vi "X-Y-Z-Move-Pro_Api.vi"() -> ()   [LabVIEW 2019]
uses:
  <vilib>/Platform/TimedLoop/XDataNode/timing_clust.ctl
  <vilib>/Platform/TimedLoop/XDataNode/nitl_modes.ctl
  <vilib>/Platform/TimedLoop/XDataNode/wakeup.ctl
  <vilib>/platform/TimedLoop/XDataNode/XDataNode.xnode
  <vilib>/Platform/TimedLoop/XDataNode/XDNodeRunTimeDep.lvlib
panel:
  out "Waveform Chart":cluster{dbl, dbl}(graph)
  in  "Stop":bool
  out "Error Out":errorcluster
  in  "Error In":errorcluster
  in  "加速度":dbl=800.0
  in  "最高速":dbl=1150.0
  in  "X-Y-Z移動":dbl[][](array[numeric])=[[0.0, 0.0, 0.0]]
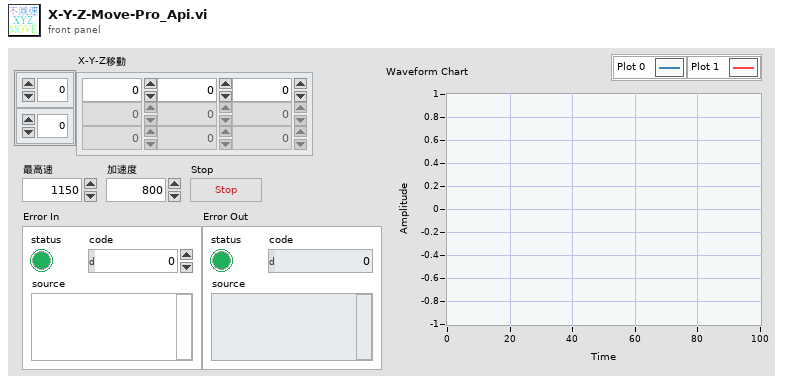
[diagram p1: front panel]
types:
  T1 = typedef "XDNodeRunTimeDep.lvlib/timing_clust.ctl" = cluster{"Expected End [f-1]":u64, "Actual End [f-1]":u64, "Finished Late? [f-1]":bool, "Expected End [i-1]":u64, "Actual End [i-1]":u64, "Finished Late? [i-1]":bool, "Expected Start [i]":u64, "Actual Start [i]":u64, "Expected Start [f]":u64, "Actual Start [f]":u64, "Source Name":string, "Structure Name":string, "Period":i64, "Deadline":i64, "Offset":i64, "Start":i64, "Priority":i32, "Timeout":i32, "Mode":T2, "Wakeup Reason":T3, "Error":errorcluster, "Source Type":string, "Secondary Source Type":string, "Global End Time":u64, "Global Start Time":u64, "Frame Duration":u64, "Iteration Duration":u64, "Assigned CPU":i32, "I/O Scan Engine Mode":u32}
  T2 = typedef "XDNodeRunTimeDep.lvlib/nitl_modes.ctl" = enum32{"No Change", "Process missed periods, maintain original phase", "Discard missed periods, maintain original phase", "Process missed periods, ignore original phase", "Discard missed periods, ignore original phase"}
  T3 = typedef "XDNodeRunTimeDep.lvlib/wakeup.ctl" = enum32{"Normal", "Aborted", "Asynchronous wakeup", "Timing source error", "Timed loop error", "Timeout"}
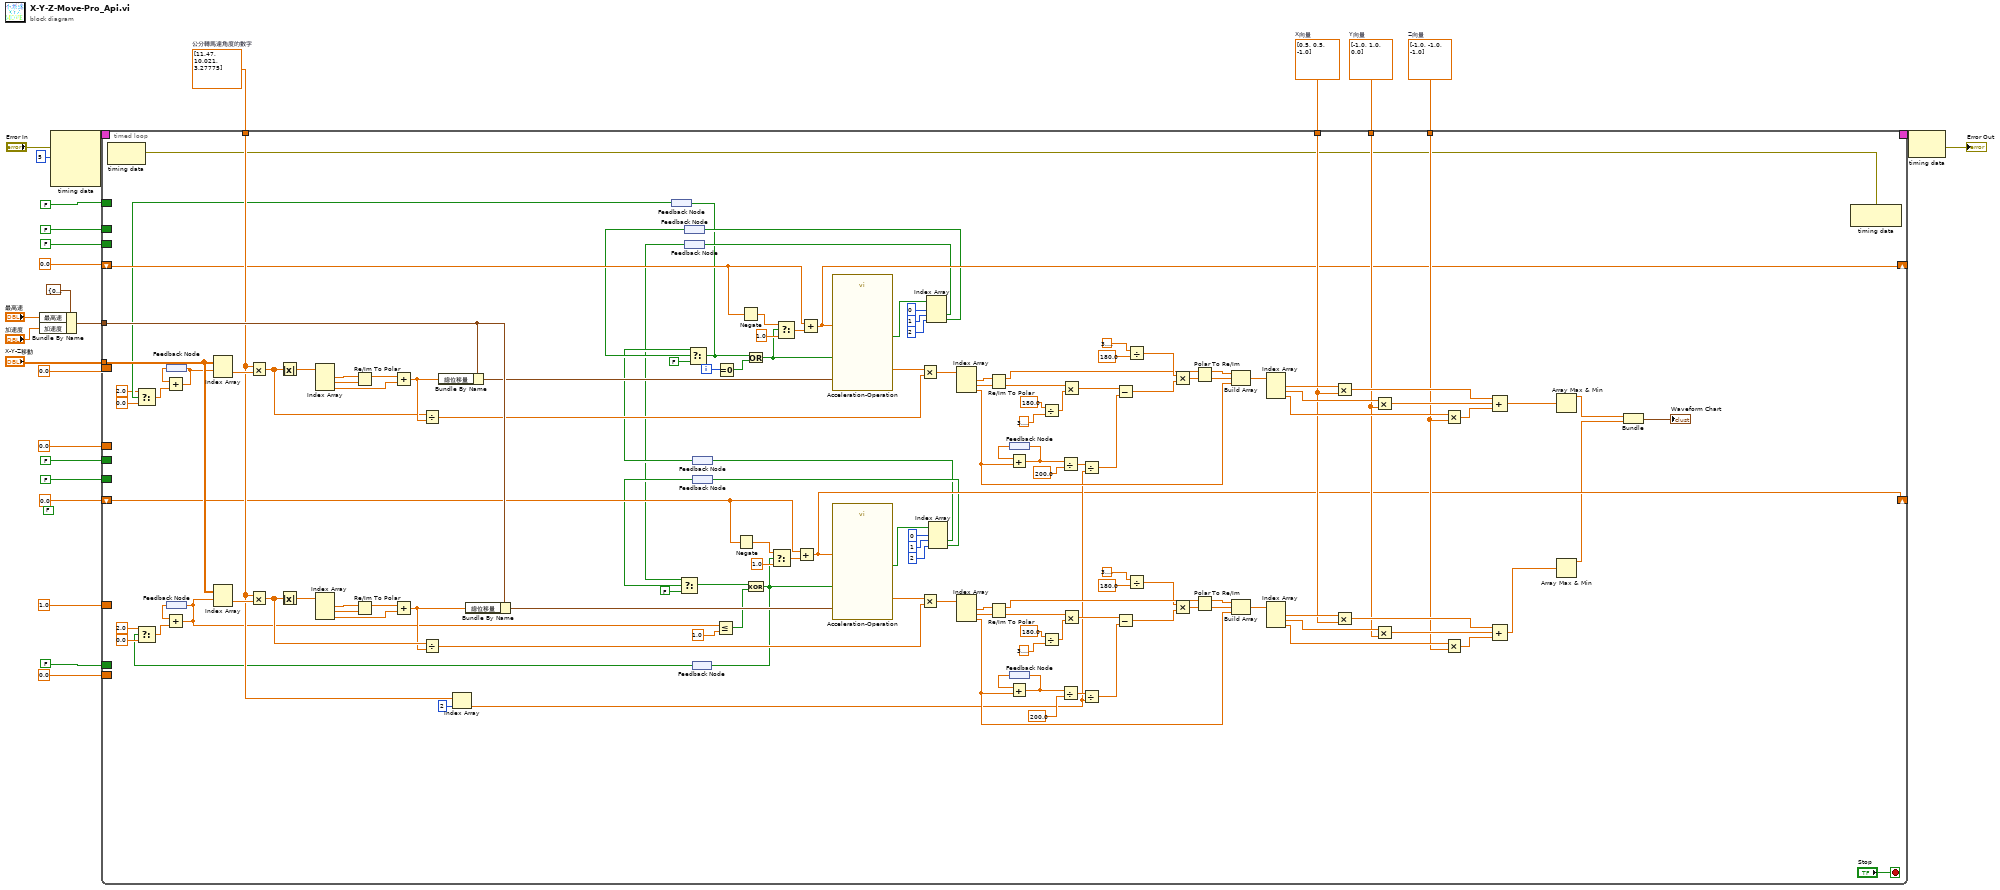
[diagram p0: block diagram]
diagram:
  (unwired) FALSE
  w15 = dbl[] [-1.0, -1.0, -1.0]  # Z向量
  w16 = dbl[] [-1.0, 1.0, 0.0]  # Y向量
  w17 = dbl[] [0.5, 0.5, -1.0]  # X向量
  w19 = dbl[] [11.47, 10.021, 3.27775]  # 公分轉馬達角度的數字
  n1 = Bundle By Name(cluster=cluster{"總位移量":dbl, "最高速":dbl, "加速度":dbl} {"總位移量"=0.0, "最高速"=0.0, "加速度"=0.0} ("計算設置"), "最高速"="最高速", "加速度"="加速度") -> (w18:cluster{"總位移量":dbl, "最高速":dbl, "加速度":dbl})
  n2 = node-c288("Error In", i64 5 ("Period")) -> (w26:T1)  [unwired: 2 in]
  n3 = timed-loop {
    timing: w26 -> [_]
    timing-out: [_] -> w25
    tunnel: "X-Y-Z移動" -> [w153]
    tunnel: w19 -> [w86]
    tunnel: w18 -> [w152]
    border: 0.0 -> [_]
    border: 0.0 -> [_]
    tunnel: w17 -> [w87]
    tunnel: w16 -> [w88]
    tunnel: w15 -> [w89]
    shift-right: [w70] -> _
    shift-left: 0.0 -> [w63]
    shift-right: [w67] -> _
    shift-left: 0.0 -> [w65]
    border: FALSE -> [_]
    border: FALSE -> [_]
    border: FALSE -> [_]
    border: FALSE -> [_]
    border: 0.0 -> [_]
    border: FALSE -> [_]
    border: 1.0 -> [_]
    border: FALSE -> [_]
    i -> [w46]
    stop <- "Stop" stop-if-true
    n4 = node-c288() -> (w82:errorcluster)  [unwired: 1 in]
    n5 = feedback #1() -> (w56:dbl)
    n6 = feedback #2() -> (w49:dbl)
    n7 = Index Array(array=w86, index=2) -> (element=w84:dbl)
    n8 = feedback #3() -> (w55:bool)
    n9 = Select(t=2.0, s=w55, f=0.0) -> (s? t:f=w57:dbl)
    n10 = Add(x=w56, y=w57) -> (x+y=w52:dbl)
    n11 = feedback-in #1(w52) -> ()
    n12 = Index Array(array=w153, index (row)=w52) -> (element=w165:dbl[])  [unwired: 1 in]
    n13 = Multiply(x=w86, y=w165) -> (x*y=w162:dbl[])
    n14 = Absolute Value(x=w162) -> (abs(x)=w163:dbl[])
    n15 = Index Array(array=w163) -> (element #1=w166:dbl, element #2=w169:dbl, element #3=w167:dbl)  [unwired: 3 in]
    n16 = Re/Im To Polar(2:w169, 3:w166) -> (1:w168:dbl)  [unwired: 1 out]
    n17 = Add(x=w168, y=w167) -> (x+y=w164:dbl)
    n18 = Divide(x=w162, y=w164) -> (x/y=w121:dbl[])
    n19 = Bundle By Name(cluster=w152, "總位移量"=w164) -> (w83:cluster{"總位移量":dbl, "最高速":dbl, "加速度":dbl})
    n20 = feedback #4() -> (w44:bool)
    n21 = feedback #5() -> (w39:bool)
    n22 = feedback #6() -> (w47:bool)
    n23 = Select(t=2.0, s=w47, f=0.0) -> (s? t:f=w48:dbl)
    n24 = Add(x=w49, y=w48) -> (x+y=w36:dbl)
    n25 = feedback-in #2(w36) -> ()
    n26 = Index Array(array=w153, index (row)=w36) -> (element=w158:dbl[])  [unwired: 1 in]
    n27 = Multiply(x=w86, y=w158) -> (x*y=w161:dbl[])
    n28 = Absolute Value(x=w161) -> (abs(x)=w160:dbl[])
    n29 = Index Array(array=w160) -> (element #1=w157:dbl, element #2=w154:dbl, element #3=w156:dbl)  [unwired: 3 in]
    n30 = Re/Im To Polar(2:w154, 3:w157) -> (1:w155:dbl)  [unwired: 1 out]
    n31 = Add(x=w155, y=w156) -> (x+y=w159:dbl)
    n32 = Divide(x=w161, y=w159) -> (x/y=w91:dbl[])
    n33 = Bundle By Name(cluster=w152, "總位移量"=w159) -> (w62:cluster{"總位移量":dbl, "最高速":dbl, "加速度":dbl})
    n34 = feedback #7() -> (w43:bool)
    n35 = Select(t=w43, s=w44, f=FALSE) -> (s? t:f=w32:bool)
    n36 = feedback-in #3(w32) -> ()
    n37 = feedback #8() -> (w40:bool)
    n38 = Select(t=w39, s=w40, f=FALSE) -> (s? t:f=w41:bool)
    n39 = Less Or Equal?(x=w36, y=1.0 ("x")) -> (x <= y?=w37:bool)
    n40 = Equal To 0?(x=w46) -> (x = 0?=w45:bool)
    n41 = Negate(x=w63) -> (-x=w72:dbl)
    n42 = Negate(x=w65) -> (-x=w66:dbl)
    n43 = Or(x=w32, y=w45) -> (x .or. y?=w33:bool)
    n44 = Exclusive Or(1:w37, 2:w41) -> (0:w35:bool)
    n45 = feedback-in #6(w35) -> ()
    n46 = Select(t=w72, s=w35, f=1.0) -> (s? t:f=w73:dbl)
    n47 = Select(t=w66, s=w33, f=1.0) -> (s? t:f=w68:dbl)
    n48 = Add(x=w63, y=w73) -> (x+y=w70:dbl)
    n49 = Add(x=w65, y=w68) -> (x+y=w67:dbl)
    n50 = call "Acceleration-Operation.vi"("Reset"=w33, "迴圈( I )"=w67, "計算設置"=w83) -> ("完成?"=w81:bool[], "速度"=w122:dbl)  [unwired: 6 in, 1 out]
    n51 = call "Acceleration-Operation.vi"("Reset"=w35, "迴圈( I )"=w70, "計算設置"=w62) -> ("完成?"=w74:bool[], "速度"=w90:dbl)  [unwired: 6 in, 1 out]
    n52 = Multiply(x=w122, y=w121) -> (x*y=w151:dbl[])
    n53 = Multiply(x=w90, y=w91) -> (x*y=w92:dbl[])
    n54 = Index Array(array=w81, index #1=0 ("index"), index #2=1 ("index"), index #3=2 ("index")) -> (element #2=w64:bool, element #3=w60:bool)  [unwired: 1 out]
    n55 = feedback-in #4(w60) -> ()
    n56 = feedback-in #5(w64) -> ()
    n57 = Index Array(array=w74, index #1=0 ("index"), index #2=1 ("index"), index #3=2 ("index")) -> (element #2=w59:bool, element #3=w61:bool)  [unwired: 1 out]
    n58 = feedback-in #7(w59) -> ()
    n59 = feedback-in #8(w61) -> ()
    n60 = Index Array(array=w151) -> (element #1=w150:dbl, element #2=w149:dbl, element #3=w132:dbl)  [unwired: 3 in]
    n61 = Index Array(array=w92) -> (element #1=w93:dbl, element #2=w94:dbl, element #3=w111:dbl)  [unwired: 3 in]
    n62 = Re/Im To Polar(2:w149, 3:w150) -> (0:w148:dbl, 1:w135:dbl)
    n63 = Re/Im To Polar(2:w94, 3:w93) -> (0:w95:dbl, 1:w108:dbl)
    n64 = feedback #9() -> (w144:dbl)
    n65 = Add(x=w144, y=w132) -> (x+y=w143:dbl)
    n66 = feedback-in #9(w143) -> ()
    n67 = feedback #10() -> (w99:dbl)
    n68 = Add(x=w99, y=w111) -> (x+y=w100:dbl)
    n69 = feedback-in #10(w100) -> ()
    n70 = Divide(x=180.0, y=3.141592653589793) -> (x/y=w145:dbl)
    n71 = Divide(x=180.0, y=3.141592653589793) -> (x/y=w98:dbl)
    n72 = Divide(x=w143, y=200.0) -> (x/y=w124:dbl)
    n73 = Divide(x=w100, y=200.0) -> (x/y=w119:dbl)
    n74 = Multiply(x=w148, y=w145) -> (x*y=w141:dbl)
    n75 = Multiply(x=w95, y=w98) -> (x*y=w102:dbl)
    n76 = Divide(x=w124, y=w84) -> (x/y=w123:dbl)
    n77 = Divide(x=w119, y=w84) -> (x/y=w120:dbl)
    n78 = Subtract(x=w141, y=w123) -> (x-y=w137:dbl)
    n79 = Subtract(x=w102, y=w120) -> (x-y=w106:dbl)
    n80 = Divide(x=3.141592653589793, y=180.0 ("x")) -> (x/y=w138:dbl)
    n81 = Divide(x=3.141592653589793, y=180.0 ("x")) -> (x/y=w105:dbl)
    n82 = Multiply(x=w138, y=w137) -> (x*y=w136:dbl)
    n83 = Multiply(x=w105, y=w106) -> (x*y=w107:dbl)
    n84 = Polar To Re/Im(2:w136, 3:w135) -> (0:w133:dbl, 1:w134:dbl)
    n85 = Polar To Re/Im(2:w107, 3:w108) -> (0:w110:dbl, 1:w109:dbl)
    n86 = Build Array(w134, w133, w132) -> (w131:dbl[])
    n87 = Build Array(w109, w110, w111) -> (w112:dbl[])
    n88 = Index Array(array=w131) -> (element #1=w130:dbl, element #2=w129:dbl, element #3=w128:dbl)  [unwired: 3 in]
    n89 = Index Array(array=w112) -> (element #1=w113:dbl, element #2=w114:dbl, element #3=w115:dbl)  [unwired: 3 in]
    n90 = Multiply(x=w130, y=w87) -> (x*y=w127:dbl[])
    n91 = Multiply(x=w113, y=w87) -> (x*y=w116:dbl[])
    n92 = Multiply(x=w129, y=w88) -> (x*y=w126:dbl[])
    n93 = Multiply(x=w114, y=w88) -> (x*y=w117:dbl[])
    n94 = Multiply(x=w128, y=w89) -> (x*y=w125:dbl[])
    n95 = Multiply(x=w115, y=w89) -> (x*y=w118:dbl[])
    n96 = Compound Arithmetic op=ADD(w127, w126, w125) -> (w31:dbl[])
    n97 = Compound Arithmetic op=ADD(w116, w117, w118) -> (w30:dbl[])
    n98 = Array Max & Min(array=w31) -> (max value=w28:dbl)  [unwired: 3 out]
    n99 = Array Max & Min(array=w30) -> (max value=w29:dbl)  [unwired: 3 out]
    n100 = Bundle(w28, w29) -> (→"Waveform Chart":cluster{dbl, dbl})  [unwired: 1 in]
    n101 = node-c288(w82) -> ()  [unwired: 1 out]
  }
  n102 = node-c288(w25) -> (→"Error Out":errorcluster)
